vi "Resting.vi"() -> (0 "Terminate VI":bool)   [LabVIEW 2020]
uses:
  Traffic Signal.ctl
  Grade Gate.ctl
  PedX Signal.ctl
  Global Indicators.vi
panel:
  out "NS-4 OUTPUT":T1
  out "NS-3 OUTPUT":T1
  out "NS-2 OUTPUT":T1
  out "NS-1 OUTPUT":T1
  out "WE-4 OUTPUT":T1
  out "WE-3 OUTPUT":T1
  out "WE-2 OUTPUT":T1
  out "WE-1 OUTPUT":T1
  out "Grade Gate West OUTPUT":T2
  out "Grade Gate East OUTPUT":T2
  out "Northbound OUTPUT":T3
  out "Eastbound OUTPUT":T3
  out "Southbound OUTPUT":T3
  out "Westbound OUTPUT":T3
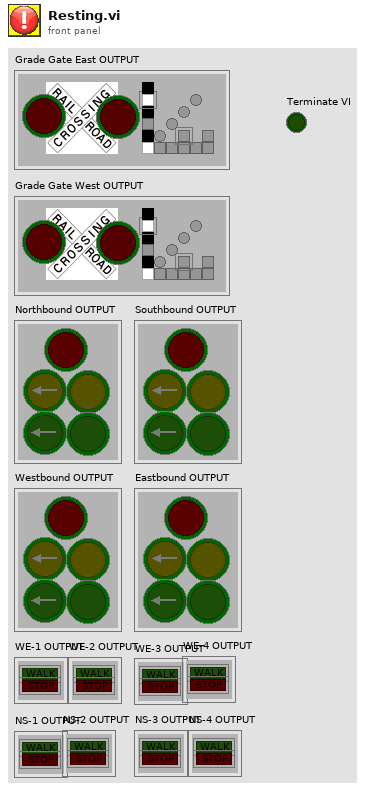
[diagram p1: front panel]
types:
  T1 = typedef "PedX Signal.ctl" = cluster{"PedX Walk":bool, "PedX Stop":bool}
  T2 = typedef "Grade Gate.ctl" = cluster{"UP 2":bool, "Pivot":bool, "UP 3":bool, "UP 4":bool, "UP 5":bool, "UP 6":bool, "DOWN 2":bool, "DOWN 3":bool, "DOWN 4":bool, "DOWN 5":bool, "DOWN 6":bool, "DOWN 7":bool, "DOWN 8":bool, "SIDE 2":bool, "SIDE 3":bool, "SIDE 4":bool, "SIDE 5":bool, "Blinky 2":bool, "Blinky 1":bool}
  T3 = typedef "Traffic Signal.ctl" = cluster{"Red Light":bool, "Yellow Light":bool, "Green Light":bool, "Yellow Turn":bool, "Green Turn":bool}
  T4 = enum16{"Start Loop", "Phase 1", "Blink 1", "Blink 2"}
  T5 = typedef "Reset.ctl" = bool
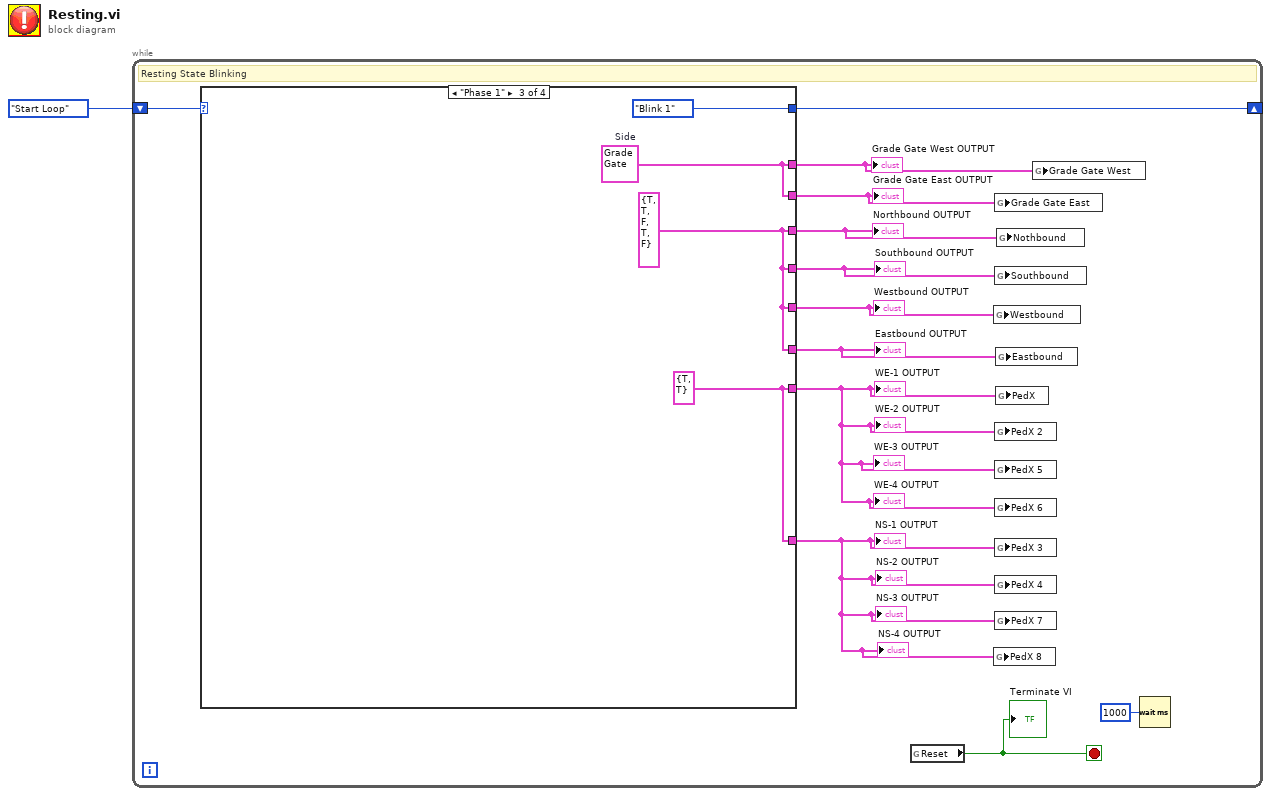
[diagram p0: block diagram]
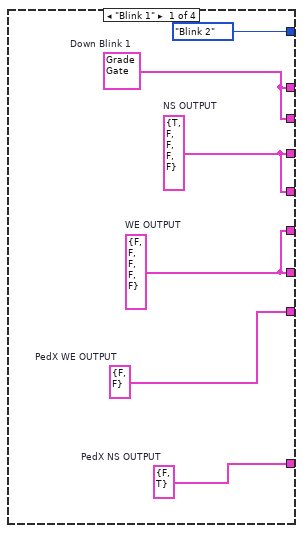
[diagram p2: hidden frame]
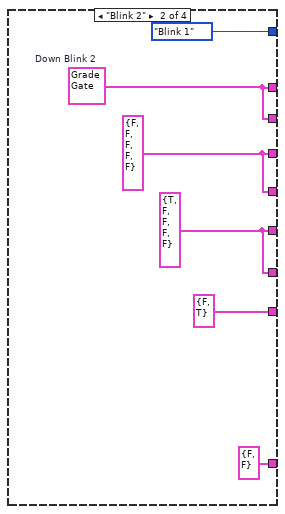
[diagram p3: hidden frame]
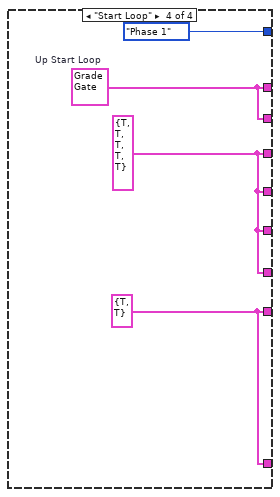
[diagram p4: hidden frame]
diagram:
  n1 = while {
    shift-right: [w11] -> _
    shift-left: T4."Start Loop" -> [w12]
    stop <- w2 stop-if-true
    # "Resting State Blinking"
    n2 = case shown="\"Phase 1\"" w12 {
      tunnel: [T4."Blink 2" T4."Blink 1" T4."Blink 1" T4."Phase 1"] -> w11
      tunnel: [w15 w20 w29 w32] -> w10
      tunnel: [w15 w20 w29 w32] -> w3
      tunnel: [w19 w24 w28 w31] -> w4
      tunnel: [w18 w23 w28 w31] -> w7
      tunnel: [w18 w23 w28 w31] -> w6
      tunnel: [w19 w24 w28 w31] -> w5
      tunnel: [w17 T1 {"PedX Walk"=FALSE, "PedX Stop"=TRUE} ("WE-1 OUTPUT") w27 w30] -> w8
      tunnel: [w16 T1 {"PedX Walk"=FALSE, "PedX Stop"=FALSE} ("WE-1 OUTPUT") w27 w30] -> w9
      frame "Blink 1" {
        w16 = T1 {"PedX Walk"=FALSE, "PedX Stop"=TRUE}  # PedX NS OUTPUT
        w18 = T3 {"Red Light"=FALSE, "Yellow Light"=FALSE, "Green Light"=FALSE, "Yellow Turn"=FALSE, "Green Turn"=FALSE}  # WE OUTPUT
        w17 = T1 {"PedX Walk"=FALSE, "PedX Stop"=FALSE}  # PedX WE OUTPUT
        w19 = T3 {"Red Light"=TRUE, "Yellow Light"=FALSE, "Green Light"=FALSE, "Yellow Turn"=FALSE, "Green Turn"=FALSE}  # NS OUTPUT
        w15 = T2 {"UP 2"=TRUE, "Pivot"=FALSE, "UP 3"=FALSE, "UP 4"=TRUE, "UP 5"=TRUE, "UP 6"=TRUE, "DOWN 2"=TRUE, "DOWN 3"=TRUE, "DOWN 4"=TRUE, "DOWN 5"=TRUE, "DOWN 6"=TRUE, "DOWN 7"=FALSE, "DOWN 8"=TRUE, "SIDE 2"=FALSE, "SIDE 3"=FALSE, "SIDE 4"=FALSE, "SIDE 5"=FALSE, "Blinky 2"=TRUE, "Blinky 1"=FALSE}  # Down Blink 1
      }
      frame "Blink 2" {
        w23 = T3 {"Red Light"=TRUE, "Yellow Light"=FALSE, "Green Light"=FALSE, "Yellow Turn"=FALSE, "Green Turn"=FALSE} ("Northbound OUTPUT")
        w24 = T3 {"Red Light"=FALSE, "Yellow Light"=FALSE, "Green Light"=FALSE, "Yellow Turn"=FALSE, "Green Turn"=FALSE} ("Northbound OUTPUT")
        w20 = T2 {"UP 2"=TRUE, "Pivot"=FALSE, "UP 3"=FALSE, "UP 4"=TRUE, "UP 5"=TRUE, "UP 6"=TRUE, "DOWN 2"=TRUE, "DOWN 3"=TRUE, "DOWN 4"=TRUE, "DOWN 5"=TRUE, "DOWN 6"=TRUE, "DOWN 7"=TRUE, "DOWN 8"=FALSE, "SIDE 2"=FALSE, "SIDE 3"=FALSE, "SIDE 4"=FALSE, "SIDE 5"=FALSE, "Blinky 2"=FALSE, "Blinky 1"=TRUE}  # Down Blink 2
      }
      frame "Phase 1" {
        w27 = T1 {"PedX Walk"=TRUE, "PedX Stop"=TRUE} ("WE-1 OUTPUT")
        w28 = T3 {"Red Light"=TRUE, "Yellow Light"=TRUE, "Green Light"=FALSE, "Yellow Turn"=TRUE, "Green Turn"=FALSE} ("Northbound OUTPUT")
        w29 = T2 {"UP 2"=TRUE, "Pivot"=FALSE, "UP 3"=FALSE, "UP 4"=TRUE, "UP 5"=TRUE, "UP 6"=TRUE, "DOWN 2"=FALSE, "DOWN 3"=FALSE, "DOWN 4"=FALSE, "DOWN 5"=FALSE, "DOWN 6"=FALSE, "DOWN 7"=FALSE, "DOWN 8"=FALSE, "SIDE 2"=TRUE, "SIDE 3"=TRUE, "SIDE 4"=TRUE, "SIDE 5"=TRUE, "Blinky 2"=FALSE, "Blinky 1"=FALSE}  # Side
      }
      frame "Start Loop" {
        w30 = T1 {"PedX Walk"=TRUE, "PedX Stop"=TRUE} ("WE-1 OUTPUT")
        w31 = T3 {"Red Light"=TRUE, "Yellow Light"=TRUE, "Green Light"=TRUE, "Yellow Turn"=TRUE, "Green Turn"=TRUE} ("Northbound OUTPUT")
        w32 = T2 {"UP 2"=FALSE, "Pivot"=FALSE, "UP 3"=TRUE, "UP 4"=FALSE, "UP 5"=FALSE, "UP 6"=FALSE, "DOWN 2"=FALSE, "DOWN 3"=FALSE, "DOWN 4"=FALSE, "DOWN 5"=FALSE, "DOWN 6"=FALSE, "DOWN 7"=FALSE, "DOWN 8"=FALSE, "SIDE 2"=FALSE, "SIDE 3"=FALSE, "SIDE 4"=FALSE, "SIDE 5"=FALSE, "Blinky 2"=FALSE, "Blinky 1"=FALSE}  # Up Start Loop
      }
    }
    "Westbound OUTPUT" <- w6
    "Southbound OUTPUT" <- w5
    "Eastbound OUTPUT" <- w7
    "Northbound OUTPUT" <- w4
    "Grade Gate East OUTPUT" <- w3
    "Grade Gate West OUTPUT" <- w10
    "WE-1 OUTPUT" <- w8
    "WE-2 OUTPUT" <- w8
    "WE-3 OUTPUT" <- w8
    "WE-4 OUTPUT" <- w8
    "NS-1 OUTPUT" <- w9
    "NS-2 OUTPUT" <- w9
    "NS-3 OUTPUT" <- w9
    "NS-4 OUTPUT" <- w9
    n3 = global read "Global Indicators.vi" "Reset"() -> (w2:T5)
    "Terminate VI" <- w2
    n4 = global write "Global Indicators.vi" "Westbound"(w6) -> ()
    n5 = global write "Global Indicators.vi" "PedX 8"(w9) -> ()
    n6 = global write "Global Indicators.vi" "Grade Gate East"(w3) -> ()
    n7 = global write "Global Indicators.vi" "Southbound"(w5) -> ()
    n8 = global write "Global Indicators.vi" "PedX 2"(w8) -> ()
    n9 = global write "Global Indicators.vi" "PedX 5"(w8) -> ()
    n10 = global write "Global Indicators.vi" "PedX 6"(w8) -> ()
    n11 = global write "Global Indicators.vi" "PedX 3"(w9) -> ()
    n12 = global write "Global Indicators.vi" "PedX 4"(w9) -> ()
    n13 = global write "Global Indicators.vi" "PedX 7"(w9) -> ()
    n14 = global write "Global Indicators.vi" "Eastbound"(w7) -> ()
    n15 = global write "Global Indicators.vi" "PedX"(w8) -> ()
    n16 = global write "Global Indicators.vi" "Nothbound"(w4) -> ()
    n17 = global write "Global Indicators.vi" "Grade Gate West"(w10) -> ()
    n18 = Wait (ms)(milliseconds to wait=u32 1000) -> ()  [unwired: 1 out]
  }
